vi "Grader Main.vi"   [LabVIEW 2015]
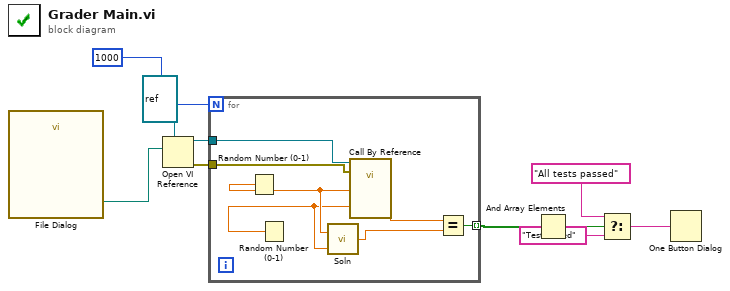
[diagram p0: block diagram]
diagram:
  n1 = call "File Dialog"() -> ("selected path"=w7:path)  [unwired: 12 in, 3 out]
  n2 = Open VI Reference(type specifier VI Refnum (for type only)=refnum<vi> refnum, vi path=w7) -> (vi reference=w9:refnum<vi>, error out=w8:errorcluster)  [unwired: 4 in]
  n3 = for {
    N: 1000 -> [_]
    tunnel: w9 -> [w17]
    tunnel: w8 -> [w16]
    tunnel: [w11] -> w5 mode=indexing
    n4 = Random Number (0-1)() -> (number: 0 to 1=w14:dbl)
    n5 = Random Number (0-1)() -> (number: 0 to 1=w13:dbl)
    n6 = call "Soln.vi"("Num2"=w13, "Num1"=w14) -> ("Sum"=w12:dbl)
    n7 = call-by-ref "?"(reference=w17, error in=w16, "Num2"=w13, "Num1"=w14) -> ("Sum"=w15:dbl)  [unwired: 2 out]
    n8 = Equal?(x=w15, y=w12) -> (x = y?=w11:bool)
  }
  n9 = And Array Elements(Boolean array=w5) -> (logical AND=w4:bool)
  n10 = Select(t="All tests passed", s=w4, f="Tests failed") -> (s? t:f=w2:string)
  n11 = One Button Dialog(message=w2) -> ()  [unwired: 1 in, 1 out]
